vi "EncodersGyroToXY.vi"(6 "Reset":bool, 9 "Angle (degrees)":dbl, 10 "Right Distance":dbl, 11 "Left Distance":dbl) -> (3 "Location":cluster{dbl, dbl})   [LabVIEW 2017]
doc: "Uses gyro and encoder data with kinematics to find XY location of robot.\n\nThe graph and locations to keep is just for visualazation purposes. It might want to be removed because of the extra processing power."
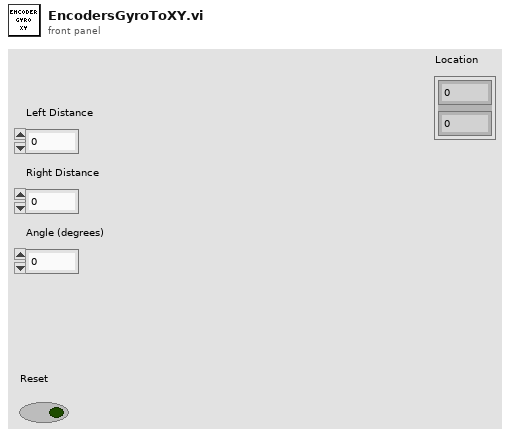
[diagram p1: front panel]
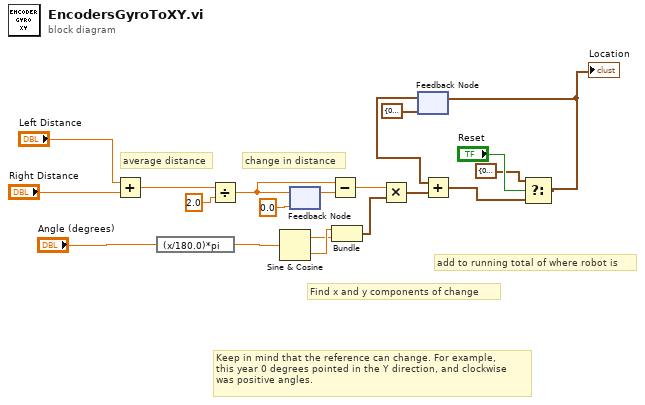
[diagram p0: block diagram]
diagram:
  # "Keep in mind that the reference can change. For example,\nthis year 0 degrees pointed in the Y direction, and clockwise\nwas positive angles."
  # "add to running total of where robot is"
  # "Find x and y components of change"
  # "change in distance"
  # "average distance"
  n1 = Add(x="Left Distance", y="Right Distance") -> (x+y=w7:dbl)
  n2 = expression code="(x/180.0)*pi" ("degrees to radians")("Angle (degrees)") -> (w17:dbl)
  n3 = Divide(x=w7, y=2.0) -> (x/y=w6:dbl)
  n4 = Sine & Cosine(0:w17) -> (1:w15:dbl, 2:w16:dbl)
  n5 = feedback #1(0.0) -> (w20:dbl)
  n6 = feedback-in #1(w6) -> ()
  n7 = Subtract(x=w6, y=w20) -> (x-y=w13:dbl)
  n8 = Bundle(w16, w15) -> (w14:cluster{dbl, dbl})  [unwired: 1 in]
  n9 = Multiply(x=w13, y=w14) -> (x*y=w12:cluster{dbl, dbl})
  n10 = feedback #2(cluster{dbl, dbl} {0.0, 0.0}) -> (w11:cluster{dbl, dbl})
  n11 = Add(x=w11, y=w12) -> (x+y=w2:cluster{dbl, dbl})
  n12 = Select(t=cluster{dbl, dbl} {0.0, 0.0}, s="Reset", f=w2) -> (s? t:f=w3:cluster{dbl, dbl})
  "Location" <- w3
  n13 = feedback-in #2(w3) -> ()
